vi "Z Sample Stage Control.vi"(7 "Calling VI Ref":refnum<vi>) -> ()   [LabVIEW 2020]
uses:
  <vilib>/Utility/miscctls.llb/LVPointTypeDef.ctl
  Hardware Configuration/Hardware Configuration Controls/Device Type.ctl
  Hardware Configuration/Hardware Configuration Controls/Device Function.ctl
  Device Library/Stages/Stages Controls/Stage Actions.ctl
panel:
  in  "Step 8":bool
  in  "Step 7":bool
  in  "Step 6":bool
  in  "Step 5":bool
  in  "Step 4":bool
  in  "Step 3":bool
  in  "Step 2":bool
  in  "Step 1":bool
  in  "Stage Down":bool
  in  "Stage Up":bool
  in  "Position (µm)":dbl format="%#.3g"
  in  "Step Size (µm)":dbl=0.1
  in  "Quit":bool
  # "Preset Step Sizes"
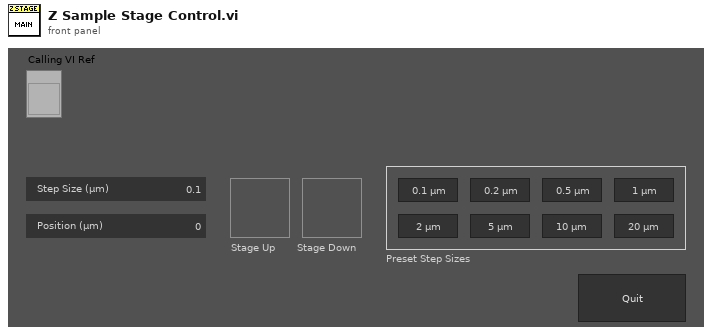
[diagram p1: front panel]
types:
  T1 = enum16{"Always On", "Always Off", "Off While Running"}
  T2 = typedef "LVPointTypeDef.ctl" = cluster{"Horizontal":i16, "Vertical":i16}
  T3 = typedef "Device Function.ctl" = enum16{"Primary", "Secondary", "Overview", "Wide Field Drift Correction", "642 nm Excitation", "560 nm Excitation", "940 nm Excitation", "546 nm Excitation", "488 nm Excitation", "405 nm Excitation", "Objective Drift Correction", "4Pi Objective Lock", "Objective XY", "Objective Z", "Sample XY", "Sample Coarse Z", "Sample Z", "4Pi Lower", "4Pi Upper", "Mojo", "Adj Cavity", "Line Scanning", "Alert"}
  T4 = typedef "Device Type.ctl" = enum16{"AOTF", "Camera", "Deformable Mirror", "Laser", "Microscope Base", "Shutter", "Stage", "Waveform", "FPGA", "Email", "Filter Wheel", "Spinning Disk"}
  T5 = typedef "Stage Actions.ctl" = enum16{"Get Position", "MVR", "MOVE", "HALT", "ONTARGET", "ERROR", "REFERENCE", "INIT", "VELOCITY", "STATUS", "EXIT", "HOME", "ZEROPOS", "NANOPOS", "ANALOG", "QUIT"}
  T6 = enum32{"Invalid", "Standard", "Closed", "Hidden", "Minimized", "Maximized"}
  T7 = typedef "LVRectTypeDef.ctl" = cluster{"Left":i16, "Top":i16, "Right":i16, "Bottom":i16}
  T8 = typedef "LVBoundsTypeDef.ctl" = cluster{"Width":u32, "Height":u32}
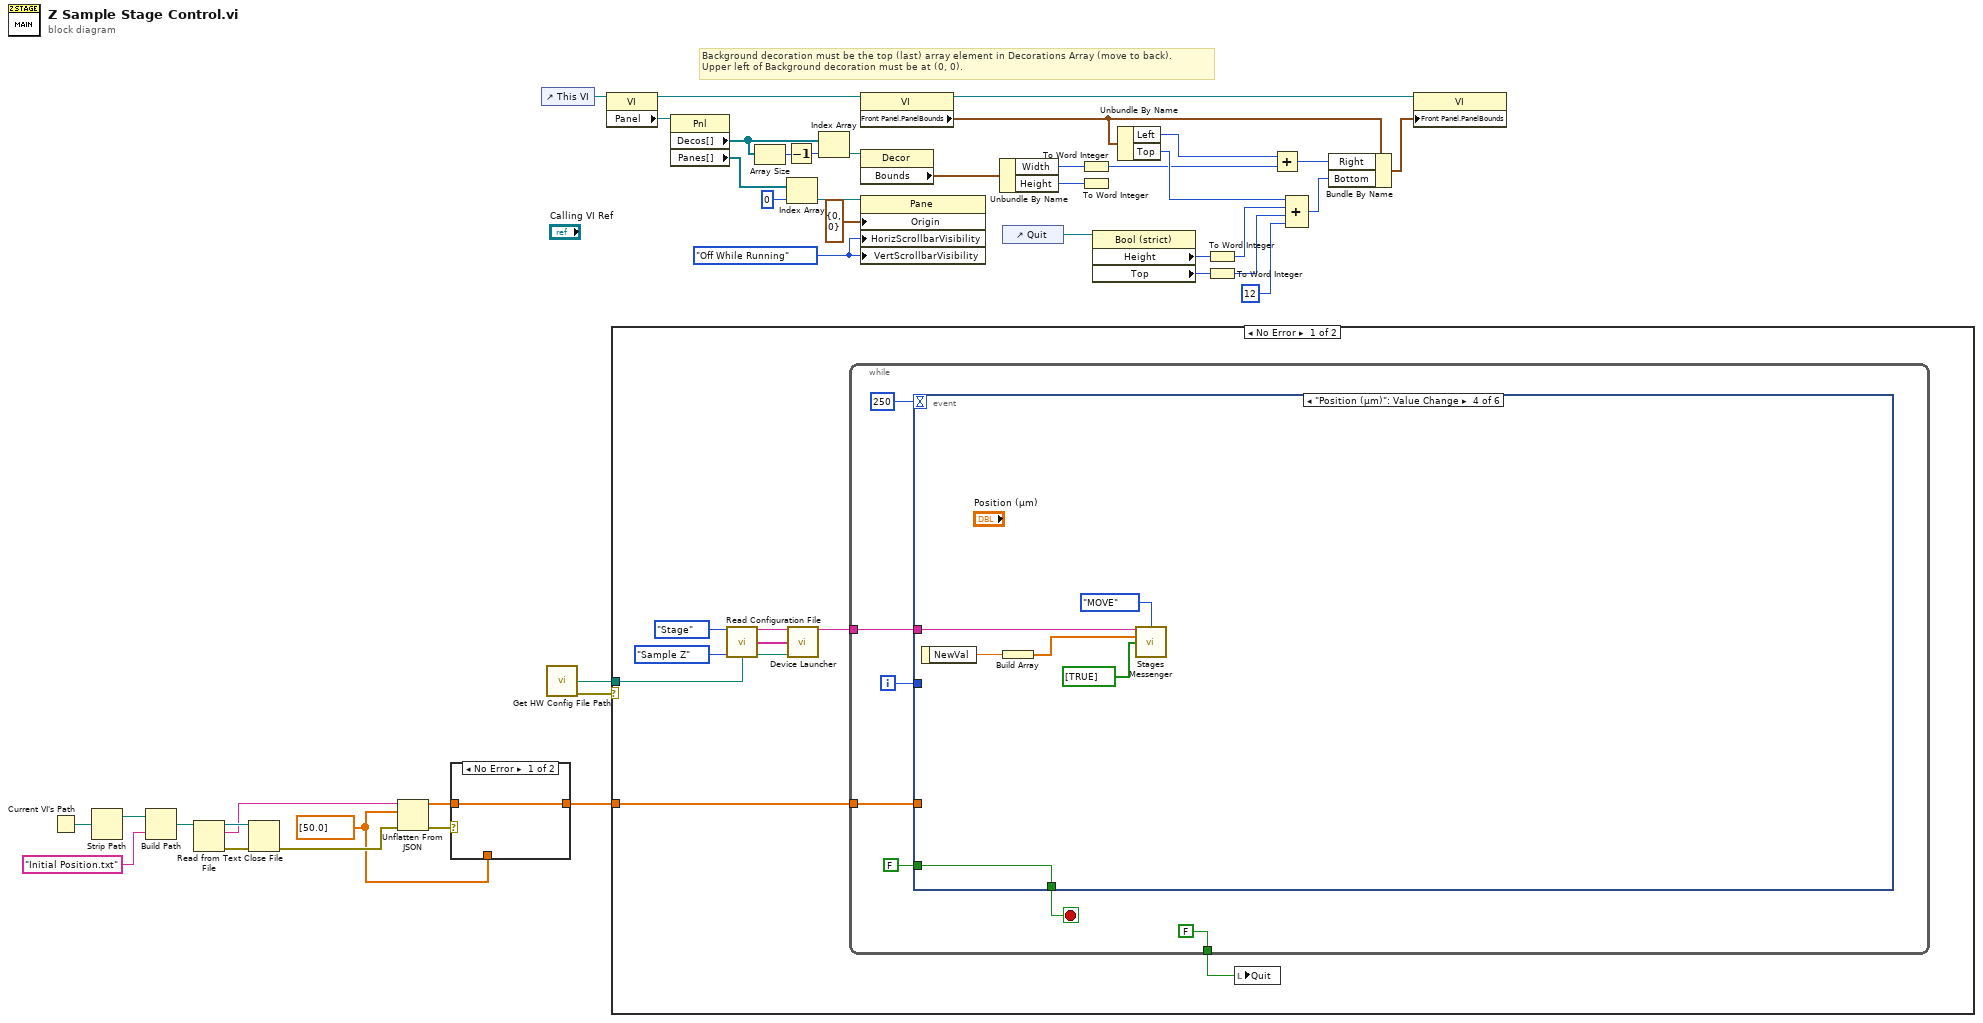
[diagram p0: block diagram]
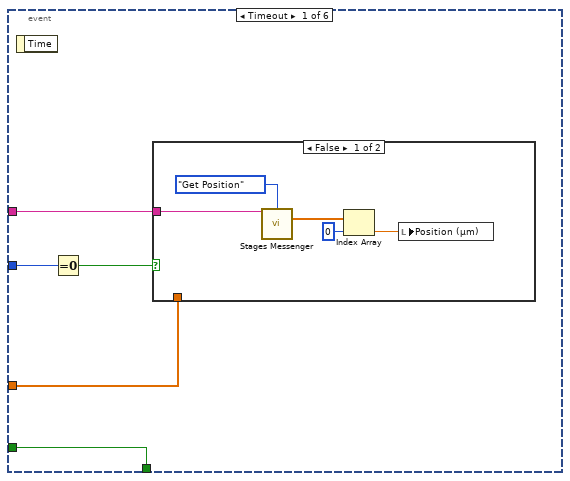
[diagram p3: hidden frame]
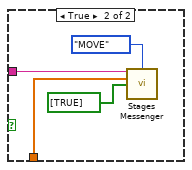
[diagram p4: hidden frame]
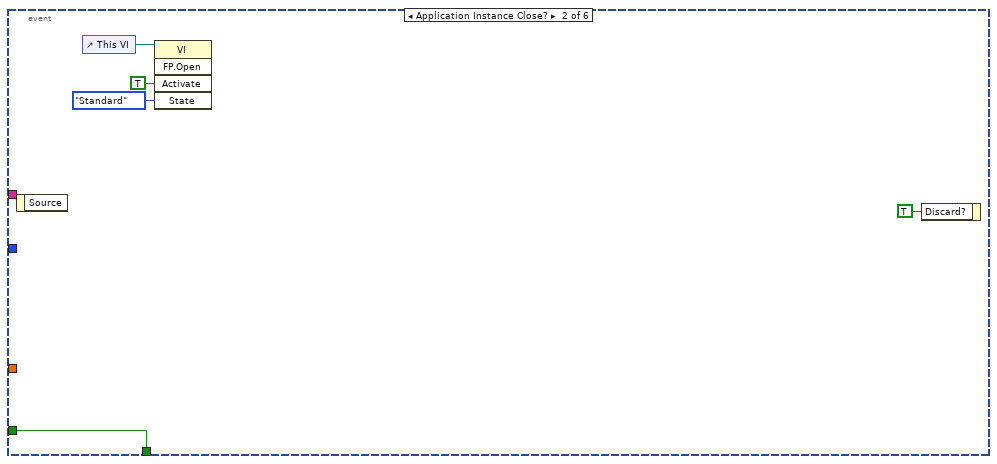
[diagram p5: hidden frame]
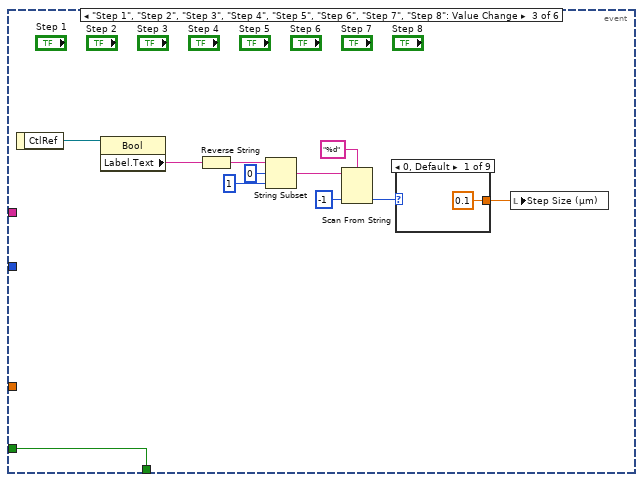
[diagram p6: hidden frame]
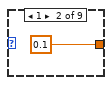
[diagram p7: hidden frame]
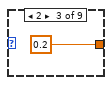
[diagram p8: hidden frame]
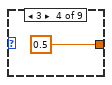
[diagram p9: hidden frame]
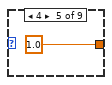
[diagram p10: hidden frame]
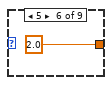
[diagram p11: hidden frame]
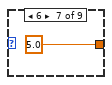
[diagram p12: hidden frame]
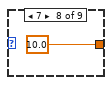
[diagram p13: hidden frame]
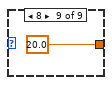
[diagram p14: hidden frame]
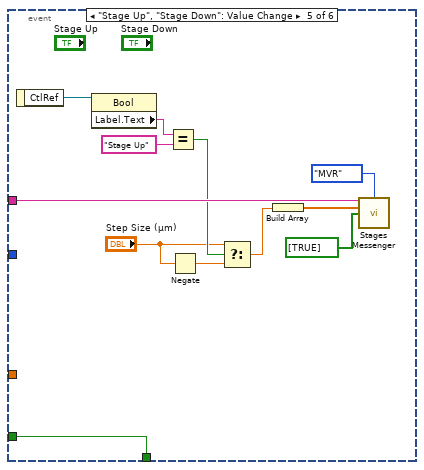
[diagram p15: hidden frame]
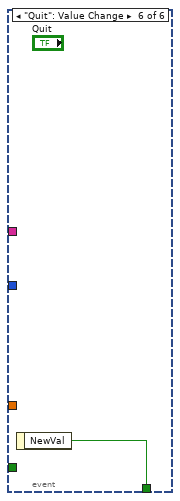
[diagram p16: hidden frame]
diagram:
  w2 = dbl[] [50.0]
  w24 = T1."Off While Running" ("Vertical Scrollbar Visibility")
  # "Background decoration must be the top (last) array element in Decorations Array (move to back).\nUpper left of Background decoration must be at (0, 0)."
  n1 = Current VI's Path() -> (path=w12:path)
  n2 = Strip Path(path=w12) -> (stripped path=w11:path)  [unwired: 1 out]
  n3 = Build Path(base path=w11, name or relative path="Initial Position.txt") -> (appended path=w9:path)
  n4 = Read from Text File(file (use dialog)=w9) -> (refnum out=w8:refnum<file>, text=w6:string, error out=w7:errorcluster)  [unwired: 3 in, 1 out]
  n5 = Close File(refnum=w8, error in=w7) -> (error out=w5:errorcluster)  [unwired: 1 out]
  n6 = Unflatten From JSON(JSON string=w6, type and defaults=w2, error in (no error)=w5) -> (value=w3:dbl[], error out=w4:errorcluster)  [unwired: 4 in]
  n7 = case shown="No Error" w4 {
    tunnel: w3 -> [w44 _]
    tunnel: [w44 w45] -> w1
    tunnel: w2 -> [_ w45]
    frame No Error {
    }
    frame Error {
    }
  }
  n8 = control-ref of="This VI"() -> (w16:refnum<vi>)
  n9 = call "Get HW Config File Path.vi"() -> ("File Path"=w42:path, "Error"=w43:errorcluster)  [unwired: 14 in]
  n10 = property class="VI"(reference=w16) -> (reference out=w25:refnum<vi>, "Panel"=w17:refnum<vi>)  [unwired: 1 in, 1 out]
  n11 = case shown="No Error" w43 {
    tunnel: w42 -> [w47 _]
    tunnel: w1 -> [w46 _]
    frame No Error {
      n12 = call "Read Configuration File.vi"("Device Type"=Device_Type."Stage", "Device Function"=Device_Function."Sample Z", "Config File Path"=w47) -> ("Unique Notifier Name"=w52:string, "Device Ports/IDs/Channels"=w54:string[], "Device Engine Path"=w53:path)  [unwired: 9 in, 1 out]
      n13 = call "Device Launcher.vi"("Notifier Name"=w52, "Device Ports/IDs/Channels"=w54, "Device Engine Path"=w53) -> ("Notifier Name"=w49:string)  [unwired: 11 in, 1 out]
      n14 = while {
        tunnel: w49 -> [w57]
        tunnel: [FALSE] -> w48
        tunnel: w46 -> [w55]
        i -> [w56]
        stop <- w59 stop-if-true
        n15 = event shown="[3] \"Position (µm)\": Value Change" {
          selector: _ -> [_ _ _ _ _ _]
          dyn-events: _ -> [_ _ _ _ _ _]
          timeout: 250 -> [_ _ _ _ _ _]
          tunnel: FALSE -> [w66 w79 w91 w106 w118 _]
          tunnel: [w66 w79 w91 w106 w118 w119] -> w59
          tunnel: w57 -> [w63 _ _ w103 w112 _]
          tunnel: w56 -> [w65 _ _ _ _ _]
          tunnel: w55 -> [w62 _ _ _ _ _]
          event Timeout {
            n16 = event-data() -> ()  [unwired: 1 in, 1 out]
            n17 = Equal To 0?(x=w65) -> (x = 0?=w64:bool)
            n18 = case shown="False" w64 {
              tunnel: w63 -> [w70 w74]
              tunnel: w62 -> [_ w72]
              frame False {
                n19 = call "Stages Messenger.vi"("Stage Notifier Name"=w70, "Actions"=Stage_Actions."Get Position") -> ("Positions"=w69:dbl[])  [unwired: 10 in, 3 out]
                n20 = Index Array(array=w69, index=0) -> (element=w67:dbl)
                n21 = local write "Position (µm)"(w67) -> ()
              }
              frame True {
                n22 = call "Stages Messenger.vi"("Stage Notifier Name"=w74, "Actions"=Stage_Actions."MOVE", "Setpoint"=w72, "Axis"=bool[] [TRUE]) -> ()  [unwired: 8 in, 4 out]
              }
            }
          }
          event Application Instance Close? {
            n23 = event-data() -> ()  [unwired: 1 in, 1 out]
            n24 = control-ref of="This VI"() -> (w76:refnum<vi>)
            n25 = invoke class="VI" method="FP.Open"(reference=w76, "Activate"=TRUE ("Activate?"), "State"=T6."Standard") -> ()  [unwired: 2 in, 5 out]
            n26 = event-data("Discard?"=TRUE) -> ()  [unwired: 1 in, 1 out]
          }
          event "Step 1", "Step 2", "Step 3", "Step 4", "Step 5", "Step 6", "Step 7", "Step 8": Value Change {
            n27 = event-data() -> ("CtlRef"=w90:refnum<vi>)  [unwired: 1 in]
            n28 = property class="Bool"(reference=w90) -> ("Label.Text"=w89:string)  [unwired: 1 in, 2 out]
            n29 = Reverse String(1:w89) -> (0:w88:string)
            n30 = String Subset(string=w88, offset (0)=0, length (rest)=1 ("length (rest)")) -> (substring=w85:string)
            n31 = Scan From String(format string="%d", input string=w85, default 1=-1 ("default value 1")) -> (output 1=w82:i32)  [unwired: 2 in, 3 out]
            n32 = case shown="0, Default" w82 {
              tunnel: [0.1 0.1 0.2 0.5 1.0 2.0 5.0 10.0 20.0] -> w81
              frame 0, Default {
              }
              frame 1 {
              }
              frame 2 {
              }
              frame 3 {
              }
              frame 4 {
              }
              frame 5 {
              }
              frame 6 {
              }
              frame 7 {
              }
              frame 8 {
              }
            }
            n33 = local write "Step Size (µm)"(w81) -> ()
          }
          event "Position (µm)": Value Change {
            n34 = event-data() -> ("NewVal"=w105:dbl)  [unwired: 1 in]
            n35 = Build Array(w105) -> (w102:dbl[])
            n36 = call "Stages Messenger.vi"("Stage Notifier Name"=w103, "Actions"=Stage_Actions."MOVE", "Setpoint"=w102, "Axis"=bool[] [TRUE]) -> ()  [unwired: 8 in, 4 out]
          }
          event "Stage Up", "Stage Down": Value Change {
            n37 = event-data() -> ("CtlRef"=w117:refnum<vi>)  [unwired: 1 in]
            n38 = property class="Bool"(reference=w117) -> ("Label.Text"=w116:string)  [unwired: 1 in, 2 out]
            n39 = Equal?(x=w116, y="Stage Up") -> (x = y?=w111:bool)
            n40 = Negate(x="Step Size (µm)") -> (-x=w109:dbl)
            n41 = Select(t="Step Size (µm)", s=w111, f=w109) -> (s? t:f=w108:dbl)
            n42 = Build Array(w108) -> (w107:dbl[])
            n43 = call "Stages Messenger.vi"("Stage Notifier Name"=w112, "Actions"=Stage_Actions."MVR", "Setpoint"=w107, "Axis"=bool[] [TRUE]) -> ()  [unwired: 8 in, 4 out]
          }
          event "Quit": Value Change {
            n44 = event-data() -> ("NewVal"=w119:bool)  [unwired: 1 in]
          }
        }
      }
      n45 = local write "Quit"(w48) -> ()
    }
    frame Error {
    }
  }
  n46 = property class="Pnl"(reference=w17) -> ("Decos[]"=w15:refnum<vi>[], "Panes[]"=w21:refnum<vi>[])  [unwired: 1 in, 2 out]
  n47 = Array Size(array=w15) -> (size(s)=w13:i32)
  n48 = Decrement(x=w13) -> (x-1=w14:i32)
  n49 = Index Array(array=w21, index=0) -> (element=w20:refnum<vi>)
  n50 = Index Array(array=w15, index=w14) -> (element=w23:refnum<vi>)
  n51 = property class="VI"(reference=w25) -> (reference out=w27:refnum<vi>, "Front Panel.PanelBounds"=w28:T7)  [unwired: 1 in, 1 out]
  n52 = property class="Decor"(reference=w23) -> ("Bounds"=w26:T8)  [unwired: 1 in, 2 out]
  n53 = property class="Pane"(reference=w20, "Origin"=T2 {"Horizontal"=0, "Vertical"=0}, "HorizScrollbarVisibility"=w24, "VertScrollbarVisibility"=w24) -> ()  [unwired: 1 in, 2 out]
  n54 = Unbundle By Name(w26) -> ("Width"=w31:u32, "Height"=w34:u32)
  n55 = control-ref of="Quit"() -> (w18:refnum<vi>)
  n56 = To Word Integer(number=w31) -> (16bit integer=w33:i16)
  n57 = To Word Integer(number=w34) -> ()  [unwired: 1 out]
  n58 = property class="Bool (strict)"(reference=w18) -> ("Height"=w36:u32, "Top"=w37:i32)  [unwired: 1 in, 2 out]
  n59 = Unbundle By Name(w28) -> ("Left"=w30:i16, "Top"=w41:i16)
  n60 = To Word Integer(number=w36) -> (16bit integer=w39:i16)
  n61 = To Word Integer(number=w37) -> (16bit integer=w40:i16)
  n62 = Add(x=w30, y=w33) -> (x+y=w32:i16)
  n63 = Compound Arithmetic op=ADD(w41, w39, w40, i16 12 ("y")) -> (w35:i16)
  n64 = Bundle By Name(cluster=w28, "Right"=w32, "Bottom"=w35) -> (w29:T7)
  n65 = property class="VI"(reference=w27, "Front Panel.PanelBounds"=w29) -> ()  [unwired: 1 in, 2 out]
